vi "PCO_GetInterfaceOutputFormat.vi"(8 "error in (no error)":errorcluster {"code" format="%x"}, 10 "wDestInterface":u16(ring)=1 items=["HD-SDI"=1], 11 "ph":u64) -> (0 "error out":errorcluster {"code" format="%x"}, 1 "wDestInterface out":u16(ring)=1 items=["HD-SDI"=1], 2 "ErrorMessage":i32 format="%x", 3 "ph out":u64, 5 "wFormat":u16(ring) items=["HDSDI_FORMAT_OUTPUT_OFF"=0, "HDSDI_FORMAT_1080P25_SINGLE_LINK_RGB"=1, "HDSDI_FORMAT_1080P50_DUAL_LINK_RGB"=3, "HDSDI_FORMAT_1080P30_SINGLE_LINK_RGB"=11, "HDSDI_FORMAT_1080P2997_SINGLE_LINK_RGB"=12, "HDSDI_FORMAT_1080P24_SINGLE_LINK_RGB"=13, "HDSDI_FORMAT_1080P2398_SINGLE_LINK_RGB"=14, "HDSDI_FORMAT_720P24_SINGLE_LINK_RGB"=23, "HDSDI_FORMAT_720P2398_SINGLE_LINK_RGB"=24])   [LabVIEW 2020, in "SDK.lvlib" / "SpecialCommandsDimax_HDSDI.lvlib"]
doc: "<b>Description:</b>\nThis function returns the current interface output format. For the pco.dimax the interface output shows the selection of the active image streaming interface. If the interface format is set to [off], then image data will be transferred through the standard interface, e.g. GigE or USB. If the interface is set to any of the predefined HD-SDI modes a continuous image data stream is output on the HD-SDI connector and the current image size setting of the camera depend on the selected HD-SDI format. Setting of ROI is not possible when HD-SDI output is enabled.\n\n<b>Supported camera type:</b>\npco.dimax with HD-SDI interface\n\n<b>Descriptor dependency:</b>\nNone"
uses:
  SpecialCommandsDimax_HDSDI.lvlib
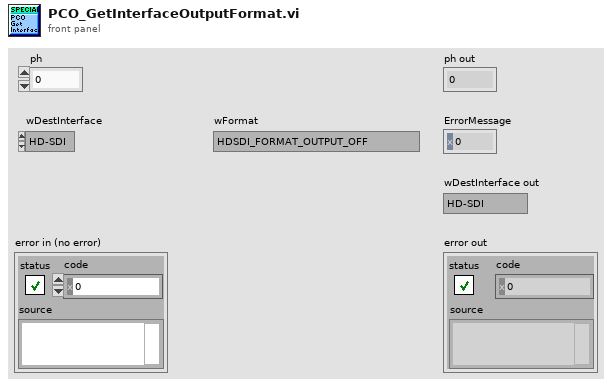
[diagram p1: front panel]
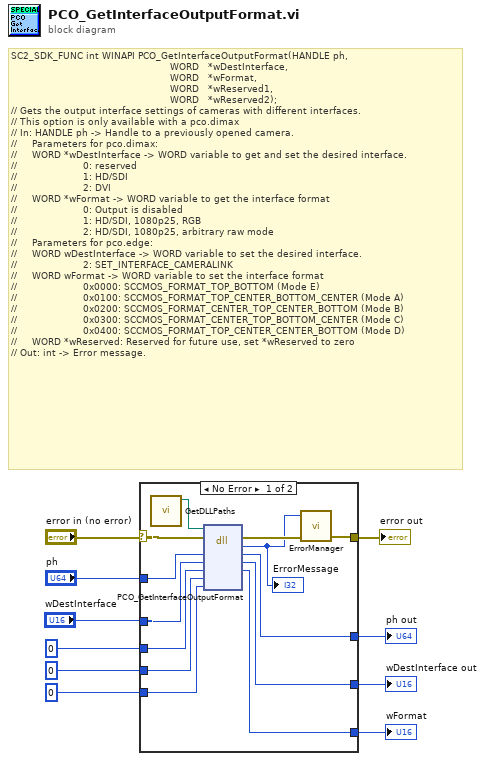
[diagram p0: block diagram]
diagram:
  # "SC2_SDK_FUNC int WINAPI PCO_GetInterfaceOutputFormat(HANDLE ph,\n                                                     WORD   *wDestInterface,\n                                                     WORD   *wFormat,\n                                                     WORD   *wReserved1,\n                                                     WORD   *wReserved2);\n// Gets the output interface settings of cameras with different interfaces.\n// This option is only available with a pco.dimax\n// In: HANDLE ph -> Handle to a previously opened camera.\n//     Parameters for pco.dimax:\n//     WORD *wDestInterface -> WORD variable to get and set the desired interface.\n//                      0: reserved\n//                      1: HD/SDI\n//                      2: DVI\n//     WORD *wFormat -> WORD variable to get the interface format\n//                      0: Output is disabled\n//                      1: HD/SDI, 1080p25, RGB\n//                      2: HD/SDI, 1080p25, arbitrary raw mode\n//     Parameters for pco.edge:\n//     WORD wDestInterface -> WORD variable to set the desired interface.\n//                      2: SET_INTERFACE_CAMERALINK\n//     WORD wFormat -> WORD variable to set the interface format\n//                      0x0000: SCCMOS_FORMAT_TOP_BOTTOM (Mode E)\n//                      0x0100: SCCMOS_FORMAT_TOP_CENTER_BOTTOM_CENTER (Mode A)\n//                      0x0200: SCCMOS_FORMAT_CENTER_TOP_CENTER_BOTTOM (Mode B)\n//                      0x0300: SCCMOS_FORMAT_CENTER_TOP_BOTTOM_CENTER (Mode C)\n//                      0x0400: SCCMOS_FORMAT_TOP_CENTER_CENTER_BOTTOM (Mode D)\n//     WORD *wReserved: Reserved for future use, set *wReserved to zero\n// Out: int -> Error message."
  n1 = case shown="No Error" "error in (no error)" {
    selector: "error in (no error)" -> [w16 w27]
    tunnel: "ph" -> [w23 w26]
    tunnel: [w22 w26] -> w9
    tunnel: [w21 w25] -> w8
    tunnel: [w20 w24] -> w7
    tunnel: u16 0 ("wReserved1") -> [w19 _]
    tunnel: u16 0 ("wReserved2") -> [w18 _]
    tunnel: [w14 w27] -> w4
    tunnel: "wDestInterface" -> [w12 w25]
    tunnel: u16 0 ("wReserved2") -> [w17 w24]
    frame No Error {
      n2 = call "GetDLLPaths.vi"() -> ("SC2_Cam_Path"=w11:path)  [unwired: 9 in, 2 out]
      n3 = dll-call lib="?" fn="PCO_GetInterfaceOutputFormat"(path in=w11, error in=w16, "ph"=w23, "wDestInterface"=w12, "wFormat"=w17, "wReserved1"=w19, "wReserved2"=w18) -> (error out=w15:errorcluster, "return type"=w13:i32, "ph"=w22:u64, "wDestInterface"=w21:u16, "wFormat"=w20:u16)  [unwired: 3 in, 1 out]
      "ErrorMessage" <- w13
      n4 = call "ErrorManager.vi"("error in (no error)"=w15, "error code"=w13) -> ("error out"=w14:errorcluster)  [unwired: 3 in]
    }
    frame Error {
    }
  }
  "ph out" <- w9
  "wDestInterface out" <- w8
  "wFormat" <- w7
  "error out" <- w4
